vi "WPILogHeaderLengthBitfields.vi"(11 "Header Length Field":u8 format="%.0x") -> (0 "Header Remainging Bytes":u8, 1 "Timestamp Length":u8, 2 "Payload Size Length":u8, 3 "Entity ID Length":u8)   [LabVIEW 2020]
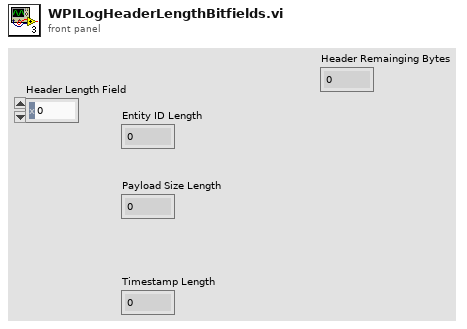
[diagram p1: front panel]
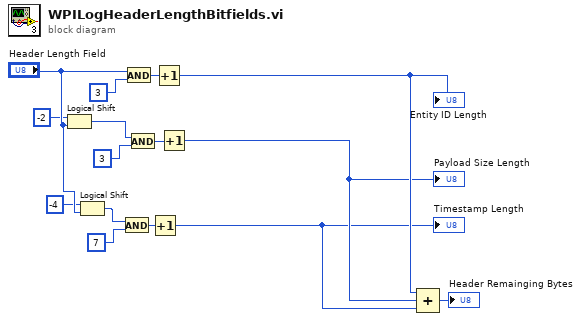
[diagram p0: block diagram]
diagram:
  n1 = Logical Shift(y=i16 -2, x="Header Length Field") -> (x << y=w9:u8)
  n2 = Logical Shift(y=i16 -4, x="Header Length Field") -> (x << y=w14:u8)
  n3 = And(x=w14, y=u8 7) -> (x .and. y?=w15:u8)
  n4 = And(x="Header Length Field", y=u8 3) -> (x .and. y?=w6:u8)
  n5 = And(x=w9, y=u8 3) -> (x .and. y?=w10:u8)
  n6 = Increment(x=w15) -> (x+1=w2:u8)
  "Timestamp Length" <- w2
  n7 = Increment(x=w6) -> (x+1=w4:u8)
  "Entity ID Length" <- w4
  n8 = Increment(x=w10) -> (x+1=w3:u8)
  "Payload Size Length" <- w3
  n9 = Compound Arithmetic op=ADD(w4, w3, w2) -> (→"Header Remainging Bytes":u8)
